vi "AuxGlobals.vi"() -> ()   [LabVIEW 2020]
panel:
  out "LETTHEREBELIGHT":bool
  in  "ShootRevRpm":dbl
  in  "ShooterSpeedMode":i32
  in  "ShootSpeedDashboard":dbl
  in  "ShooterSpeedRequest":dbl
  out "AimLimit":bool
  out "BallDetected":bool
  in  "AimLocationDemand":dbl
  in  "AimSpdDemand":dbl
  in  "AimDistance":dbl
  in  "FeedDemand":dbl
  in  "ShootDemand":dbl
  in  "BeltDemand":dbl
  in  "ShootButton":bool
  in  "RevButton":bool
  out "Intake UP":bool
  in  "IntakeSpeedDemand":dbl
  in  "BeltSpeedDemand":dbl
  in  "FeederSpeedDemand":dbl
  in  "FeederEncoderDistance":dbl
  in  "ShooterMotorOutput":dbl
  in  "ShooterRPM":dbl
  in  "ShooterSpeedDemand":dbl
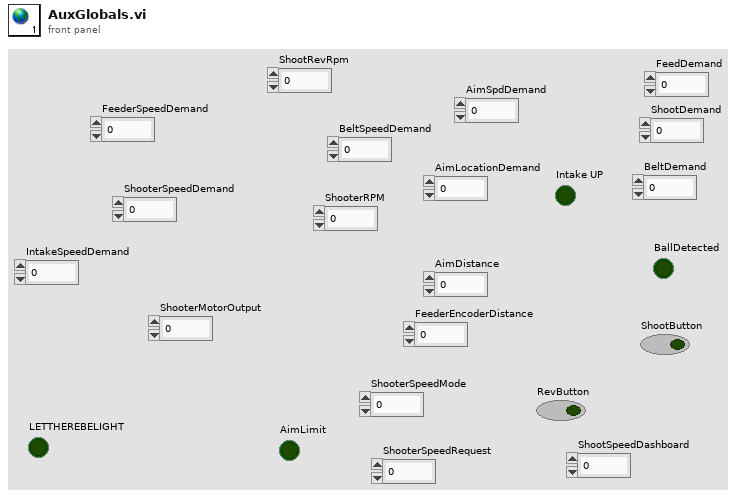
[diagram p1: front panel]
diagram:
